vi "Parser_0xE2_(SubVI).vi"(11 "String in":string) -> (1 "CheckSummGood":bool, 2 "Значение параметра":i32, 3 "Номер параметра":i32)   [LabVIEW 2017, in "LV_Unicorn.lvlib"]
uses:
  LV_Unicorn.lvlib
panel:
  out "CalcCheckSumm_U32":u32 format="%02x"
  out "ReciveCheckSumm_U32":i32 format="%x"
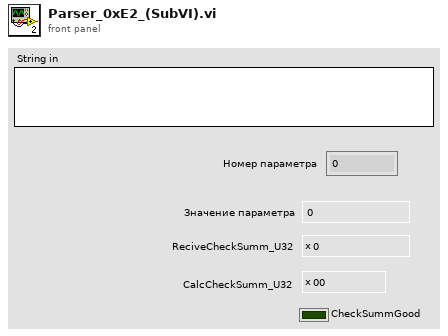
[diagram p1: front panel]
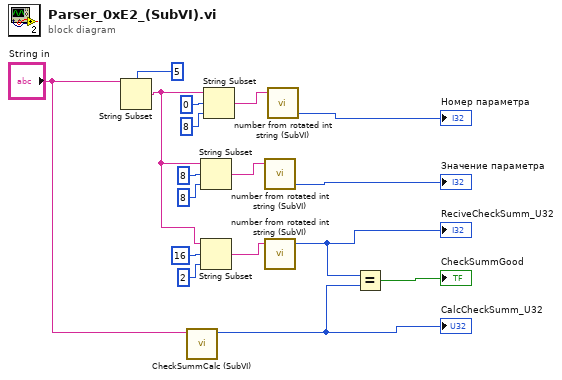
[diagram p0: block diagram]
diagram:
  n1 = String Subset(string="String in", offset (0)=5) -> (substring=w6:string)  [unwired: 1 in]
  n2 = call "CheckSummCalc (SubVI).vi"("String in"="String in") -> ("CheckSumm_U32"=w2:u32)  [unwired: 10 in]
  "CalcCheckSumm_U32" <- w2
  n3 = String Subset(string=w6, offset (0)=8, length (rest)=8 ("length (rest)")) -> (substring=w12:string)
  n4 = String Subset(string=w6, offset (0)=16, length (rest)=2 ("length (rest)")) -> (substring=w5:string)
  n5 = String Subset(string=w6, offset (0)=0, length (rest)=8 ("length (rest)")) -> (substring=w16:string)
  n6 = call "number from rotated int string (SubVI).vi"("String"=w12) -> ("int number"=→"Значение параметра":i32)  [unwired: 2 in, 2 out]
  n7 = call "number from rotated int string (SubVI).vi"("String"=w5) -> ("rotated int number"=w3:i32)  [unwired: 2 in, 2 out]
  "ReciveCheckSumm_U32" <- w3
  n8 = call "number from rotated int string (SubVI).vi"("String"=w16) -> ("int number"=→"Номер параметра":i32)  [unwired: 2 in, 2 out]
  n9 = Equal?(x=w3, y=w2) -> (x = y?=→"CheckSummGood":bool)
